vi "Add or Replace.vi"(8 "error in (no error)":errorcluster, 9 "LabVIEW Object":refnum<class>, 10 "key":string, 11 "Object Dictionary in (new)":refnum<class "objdict.lvclass">) -> (0 "error out":errorcluster, 1 "replaced Object":refnum<class>, 2 "replaced":bool, 3 "Object Dictionary out":refnum<class "objdict.lvclass">)   [LabVIEW 2015, in "objdict.lvclass"]
doc: "Adds an object to the dictionary or replaces the object assigned to the specified key. If an object is replaced, the Data Value Reference holding that object is destroyed, and the object is returned by this VI.\n\nIf faster execution is desired for add-only operations, use <b>Add.vi</b>, instead."
uses:
  objdict.lvclass
  objdict.lvclass/objdict.ctl
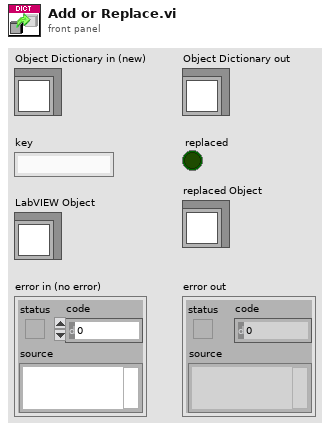
[diagram p1: front panel]
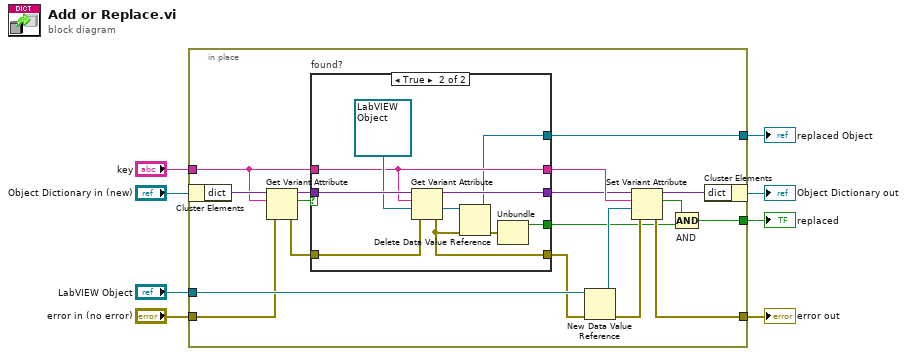
[diagram p0: block diagram]
diagram:
  n1 = in-place {
    in-place-border: [w26] -> w6
    in-place-border: "error in (no error)" -> [w19]
    in-place-border: "LabVIEW Object" -> [w23]
    in-place-border: "key" -> [w17]
    in-place-border: [w10] -> w2
    in-place-border: [w11] -> w1
    n2 = in-place-cluster #1("Object Dictionary in (new)") -> ("dict"=w20:variant)
    n3 = Get Variant Attribute(Variant=w20, name=w17, error in=w19) -> (duplicate Variant=w18:variant, found=w15:bool, error out=w16:errorcluster)  [unwired: 1 in, 1 out]
    n4 = case "found?" shown="True" w15 {
      tunnel: w18 -> [w27 w39]
      tunnel: w17 -> [w28 w35]
      tunnel: w16 -> [w29 w38]
      tunnel: [w29 w32] -> w14
      tunnel: [w28 w35] -> w13
      tunnel: [w27 w34] -> w12
      tunnel: [_ w33] -> w11
      tunnel: [_ w30] -> w9
      frame False {
      }
      frame True {
        n5 = Get Variant Attribute(Variant=w39, name=w35, default value (empty Variant)=refnum<data-value> refnum, error in=w38) -> (duplicate Variant=w34:variant, value=w37:refnum<data-value>, error out=w32:errorcluster)  [unwired: 1 out]
        n6 = Delete Data Value Reference(data value reference=w37, error in=w32) -> (data value=w33:refnum<class>, error out=w31:errorcluster)
        n7 = Unbundle(w31) -> ("status"=w30:bool)  [unwired: 2 out]
      }
    }
    n8 = New Data Value Reference(data value=w23, error in=w14) -> (data value reference=w21:refnum<data-value>, error out=w24:errorcluster)
    n9 = Set Variant Attribute(Variant=w12, name=w13, value=w21, error in=w24) -> (Variant out=w25:variant, replaced=w22:bool, error out=w26:errorcluster)
    n10 = Compound Arithmetic op=AND "AND"(w22, w9) -> (w10:bool)
    n11 = in-place-cluster #1("dict"=w25) -> (→"Object Dictionary out":refnum<class "objdict.lvclass">)
  }
  "error out" <- w6
  "replaced" <- w2
  "replaced Object" <- w1
